vi "Write Trigger Core.vi"(8 "error in (no error)":errorcluster, 10 "PV":refnum<class "PV.lvclass">, 11 "PVConnection in":refnum<class "PVConnection.lvclass">) -> (0 "error out":errorcluster, 3 "PVConnection out":refnum<class "PVConnection.lvclass">)   [LabVIEW 2015, in "CS++ProcessVariables.lvlib" / "PVConnection.lvclass"]
doc: "Publish a process variable to trigger a paramater less message."
uses:
  PVConnection.lvclass
  ProcessVariable/PV.lvclass
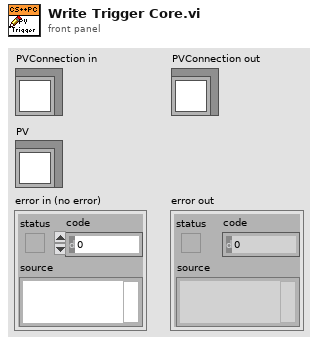
[diagram p1: front panel]
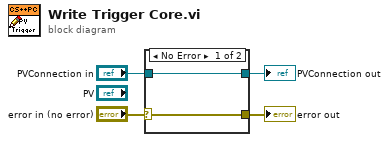
[diagram p0: block diagram]
diagram:
  n1 = case shown="No Error" "error in (no error)" {
    selector: "error in (no error)" -> [w5 w7]
    tunnel: [w5 w7] -> w4
    tunnel: [w6 w8] -> w3
    tunnel: "PVConnection in" -> [w6 w8]
    frame No Error {
    }
    frame Error {
    }
  }
  "error out" <- w4
  "PVConnection out" <- w3
